vi "PS3 Controller (SubVI).vi"(8 "error in (no error)":errorcluster, 10 "stop":bool, 11 "Refnum in":refnum<k1>) -> (0 "error out":errorcluster, 1 "Buttons":T1, 2 "Control cluster":T2, 3 "Refnum out":refnum<k1>, 5 "Arrows":i32)   [LabVIEW 2014]
uses:
  <vilib>/Utility/inputDevices.llb/joystickAcquire.vi
panel:
  # "TakeOff"
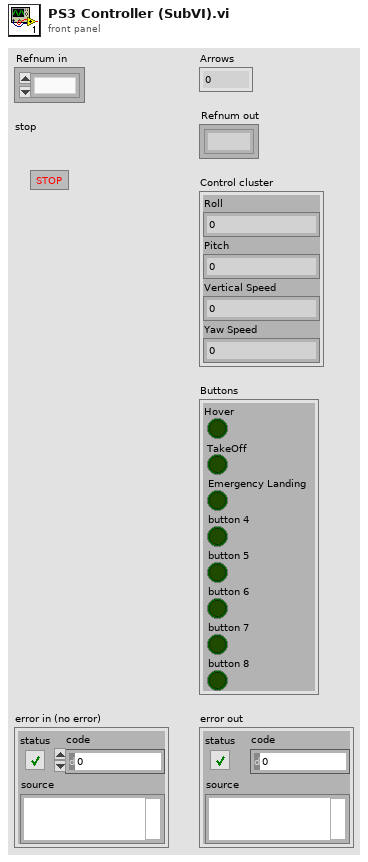
[diagram p1: front panel]
types:
  T1 = cluster{"Hover":bool, bool, "Emergency Landing":bool, "button 4":bool, "button 5":bool, "button 6":bool, "button 7":bool, "button 8":bool}
  T2 = cluster{"Roll":dbl, "Pitch":dbl, "Vertical Speed":dbl, "Yaw Speed":dbl}
  T3 = cluster{"X axis":i32, "Y axis":i32, "Z axis":i32, "X axis rotation":i32, "Y axis rotation":i32, "Z axis rotation":i32, "U axis":i32, "V axis":i32}
  T4 = cluster{"button 1":bool, "button 2":bool, "button 3":bool, "button 4":bool, "button 5":bool, "button 6":bool, "button 7":bool, "button 8":bool, "button 9":bool, "button 10":bool, "button 11":bool, "button 12":bool, "button 13":bool, "button 14":bool, "button 15":bool, "button 16":bool, "button 17":bool, "button 18":bool, "button 19":bool, "button 20":bool, "button 21":bool, "button 22":bool, "button 23":bool, "button 24":bool, "button 25":bool, "button 26":bool, "button 27":bool, "button 28":bool, "button 29":bool, "button 30":bool, "button 31":bool, "button 32":bool}
  T5 = cluster{"pov 1":i32, "pov 2":i32, "pov 3":i32, "pov 4":i32}
  T6 = cluster{"X axis":dbl, "Y axis":dbl, "Z axis":dbl, "X axis rotation":dbl, "Y axis rotation":dbl, "Z axis rotation":dbl, "U axis":dbl, "V axis":dbl}
  T7 = cluster{"button 1":bool, "button 2":bool, "button 3":bool, "button 4":bool, "button 5":bool, "button 6":bool, "button 7":bool, "button 8":bool}
  T8 = cluster{"X axis":dbl, "Y axis":dbl, "Z axis":dbl, "X axis rotation":dbl}
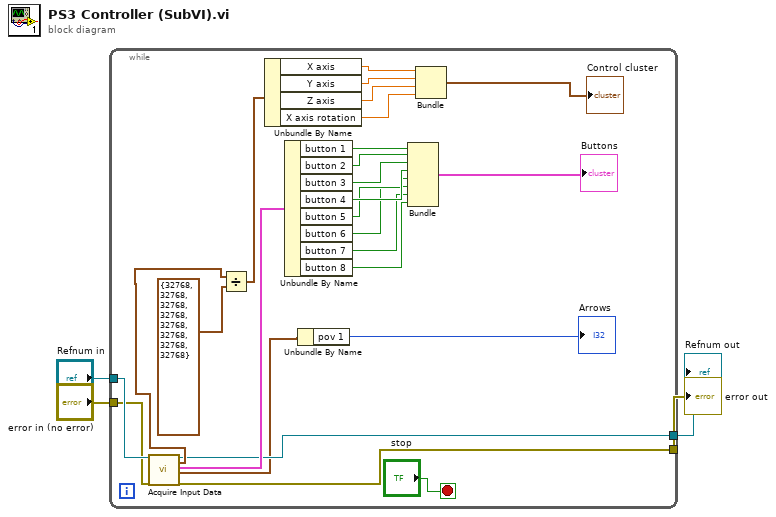
[diagram p0: block diagram]
diagram:
  n1 = while {
    tunnel: "Refnum in" -> [w29]
    tunnel: "error in (no error)" -> [w27]
    tunnel: [w22] -> w3
    tunnel: [w21] -> w4
    stop <- "stop" stop-if-true
    n2 = call-poly <vilib>:"Acquire Input Data.vi"("device ID"=w29, "error in (no error)"=w27) -> ("device ID"=w22:refnum<k1>, "axis info"=w26:T3, "button info"=w23:T4, "direction info"=w6:T5, "error out"=w21:errorcluster)  [unwired: 13 in]
    n3 = Divide(x=w26, y=T3 {"X axis"=32768, "Y axis"=32768, "Z axis"=32768, "X axis rotation"=32768, "Y axis rotation"=32768, "Z axis rotation"=32768, "U axis"=32768, "V axis"=32768}) -> (x/y=w24:T6)
    n4 = Unbundle By Name(w24) -> ("X axis"=w20:dbl, "Y axis"=w19:dbl, "Z axis"=w18:dbl, "X axis rotation"=w17:dbl)
    n5 = Unbundle By Name(w23) -> ("button 1"=w15:bool, "button 2"=w14:bool, "button 3"=w13:bool, "button 4"=w12:bool, "button 5"=w11:bool, "button 6"=w10:bool, "button 7"=w9:bool, "button 8"=w8:bool)
    n6 = Unbundle By Name(w6) -> ("pov 1"=→"Arrows":i32)
    n7 = Bundle("button 1"=w15, "button 2"=w14, "button 3"=w13, "button 4"=w12, "button 5"=w11, "button 6"=w10, "button 7"=w9, "button 8"=w8) -> (→"Buttons":T7)  [unwired: 1 in]
    n8 = Bundle("X axis"=w20, "Y axis"=w19, "Z axis"=w18, "X axis rotation"=w17) -> (→"Control cluster":T8)  [unwired: 1 in]
  }
  "error out" <- w4
  "Refnum out" <- w3
